vi "Read Measurement Data.vi"() -> (0 "Measurement Data":T1)   [LabVIEW 2012]
doc: "The Basic Serial Read and Write example performs a Serial Port Read, a Serial Port Write, or a combination of these actions. The user selects the actions (read or write) on the front panel. If both are selected, the VI will write the data first, read data, and then close the VISA session that is opened to the port. This VI will wait until the specified number of bytes is received at the port or until a termination character is read.\n\nINSTRUCTIONS:\n1) Select the serial resource and configuration parameters (baud rate, data bits, parity, stop bits, flow control).\n2) Select the operations to be performed. \n3) Connect the serial port to your device. If no device is available, perform a loopback test by doing one of the following. Short pins 2 and 3 on a RS-232 cable or short pin 4 to pin 8 and pin 5 to pin 9 on a RS-485/422 cable. \n4) Run the VI to see the data read. (The \"read string\" will match the \"string to write\" if a loopback test was performed.)\n\nNote: The parameters set for the serial port must match the parameters of the connected instrument or device. In this example, the bytes to read parameter specifies the number of bytes that the serial port reads. If there were more bytes at the port than the number specified in bytes to read, those bytes would not be read. Also, if you specify to read more bytes than the number of bytes actually read, you might receive a timeout error message.\n\nOn the block diagram, the Configure Serial Port VI sets the configuration parameters. The front panel displays the controls used to configure the basic parameters, such as baud rate, data bits, and parity. Constants configure the other parameters the user probably does not need set. After the VISA Configure Serial Port VI opens the VISA session and configures the port, the VI passes the VISA resource name to other VIs that perform operations on that VISA resource. The VISA Write function sends a command to the serial device and the VISA Read function returns data based on the command. The VISA Close function then closes the reference to the serial device. It is important to close the reference; otherwise communication through with that port through protocols other than VISA might not be possible."
uses:
  Correlator port.vi
panel:
  out "substring":string
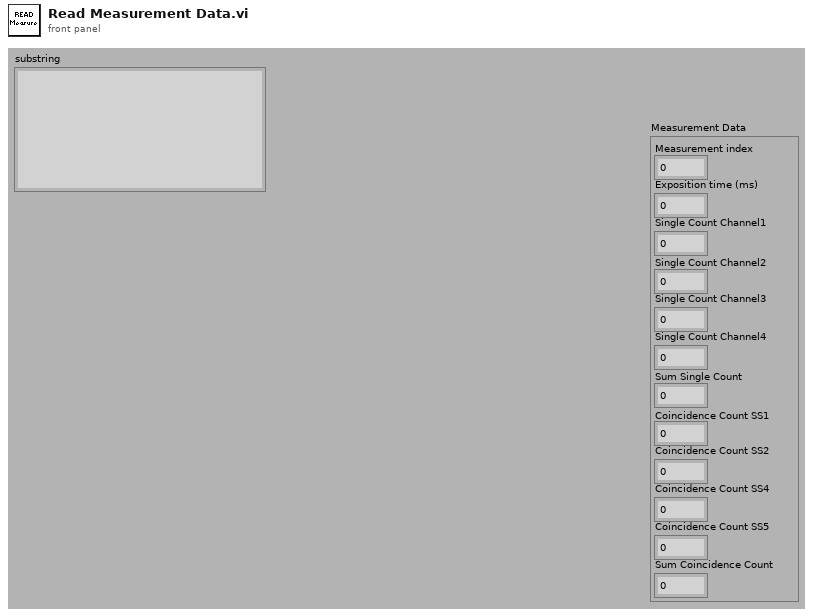
[diagram p1: front panel]
types:
  T1 = cluster{"Measurement index":i64, "Exposition time (ms)":i64, "Single Count Channel1":i64, "Single Count Channel2":i64, "Single Count Channel3":i64, "Single Count Channel4":i64, "Sum Single Count":i64, "Coincidence Count SS1":i64, "Coincidence Count SS2":i64, "Coincidence Count SS4":i64, "Coincidence Count SS5":i64, "Sum Coincidence Count":i64}
  T2 = cluster{"[0]":i64, "[1]":i64, "[2]":i64, "[3]":i64, "[4]":i64, "[5]":i64, "[6]":i64, "[7]":i64, "[8]":i64, "[9]":i64, "[10]":i64, "[11]":i64}
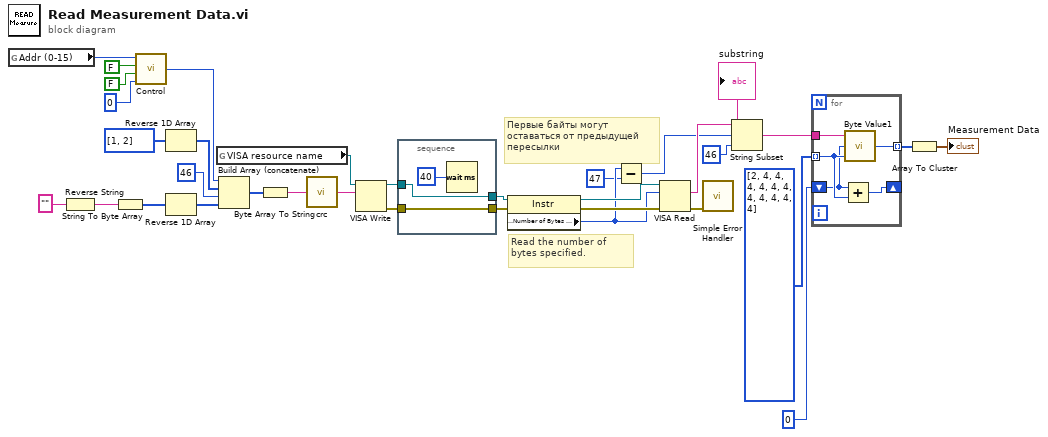
[diagram p0: block diagram]
diagram:
  # "Первые байты могут \nоставаться от предыдущей \nпересылки"
  # "Read the number of bytes specified."
  n1 = global read "Correlator port.vi" "Addr (0-15)"() -> (w7:i8)
  n2 = Reverse String(1:"" ("Data")) -> (0:w8:string)
  n3 = String To Byte Array(string=w8) -> (unsigned byte array=w13:u8[])
  n4 = call "Control.vi"("Page"=i8 0, "Error"=FALSE, "Write"=FALSE, "Addr"=w7) -> ("Control Byte"=w18:u32)
  n5 = Reverse 1D Array(array=i8[] [1, 2] ("Offset")) -> (reversed array=w16:i8[])
  n6 = Reverse 1D Array(array=w13) -> (reversed array=w12:u8[])
  n7 = global read "Correlator port.vi" "VISA resource name"() -> (w23:refnum<visa-resource-name>)
  n8 = Build Array (concatenate)(w18, w16, u8 46 ("Length"), w12) -> (w11:u32[])
  n9 = Byte Array To String(unsigned byte array=w11) -> (string=w10:string)
  n10 = call "crc.vi"("Input string"=w10) -> ("Output (with crc)"=w9:string)
  n11 = VISA Write(VISA resource name=w23, write buffer=w9) -> (VISA resource name out=w31:refnum<visa-resource-name>, error out=w33:errorcluster)  [unwired: 1 in, 1 out]
  n12 = stacked-sequence {
    tunnel: w33 -> [w36]
    tunnel: [w36] -> w32
    tunnel: w31 -> [w35]
    tunnel: [w35] -> w30
    frame #0 {
      n13 = Wait (ms)(milliseconds to wait=u32 40 ("delay before read (ms)")) -> ()  [unwired: 1 out]
    }
  }
  n14 = property class="Instr"(reference=w30, error in=w32) -> (reference out=w6:refnum<visa-resource-name>, error out=w5:errorcluster, "Serial Settings:Number of Bytes at Serial Port"=w3:u32)
  n15 = Subtract(x=w3, y=u32 47) -> (x-y=w1:u32)
  n16 = VISA Read(VISA resource name=w6, byte count=w3, error in (no error)=w5) -> (read buffer=w4:string, error out=w22:errorcluster)  [unwired: 2 out]
  n17 = call <vilib>:"Simple Error Handler.vi"("error in (no error)"=w22) -> ()  [unwired: 1 in, 8 out]
  n18 = String Subset(string=w4, offset (0)=w1, length (rest)=46 ("length (rest)")) -> (substring=w24:string)
  "substring" <- w24
  n19 = for {
    tunnel: i8[] [2, 4, 4, 4, 4, 4, 4, 4, 4, 4, 4, 4] ("Length array") -> [w40] mode=indexing
    tunnel: w24 -> [w41]
    shift-right: [w39] -> _
    shift-left: i8 0 -> [w38]
    tunnel: [w37] -> w26 mode=indexing
    n20 = Add(x=w38, y=w40) -> (x+y=w39:i8)
    n21 = call "Byte Value1.vi"("Length"=w40, "Offset"=w38, "string"=w41) -> ("Value"=w37:i64)
  }
  n22 = Array To Cluster(array=w26) -> (cluster=→"Measurement Data":T2)
